vi "Comments.Add Experiment Description.vi"(7 "error in (no error)":errorcluster, 10 "Control Experiment":refnum<class "Control Experiment.lvclass">) -> (0 "error out":errorcluster, 3 "Control Experiment out":refnum<class "Control Experiment.lvclass">)   [LabVIEW 2019, in "Control Experiment.lvclass"]
uses:
  Control Experiment.lvclass
  Control Experiment.lvclass/Control Experiment.ctl
  <userlib>/LevyLab/PLYM/YAML.lvclass
panel:
  out "Experiment Description":string
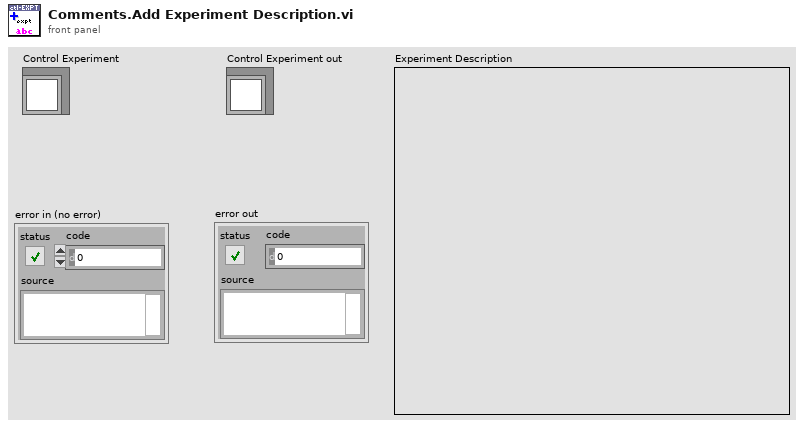
[diagram p1: front panel]
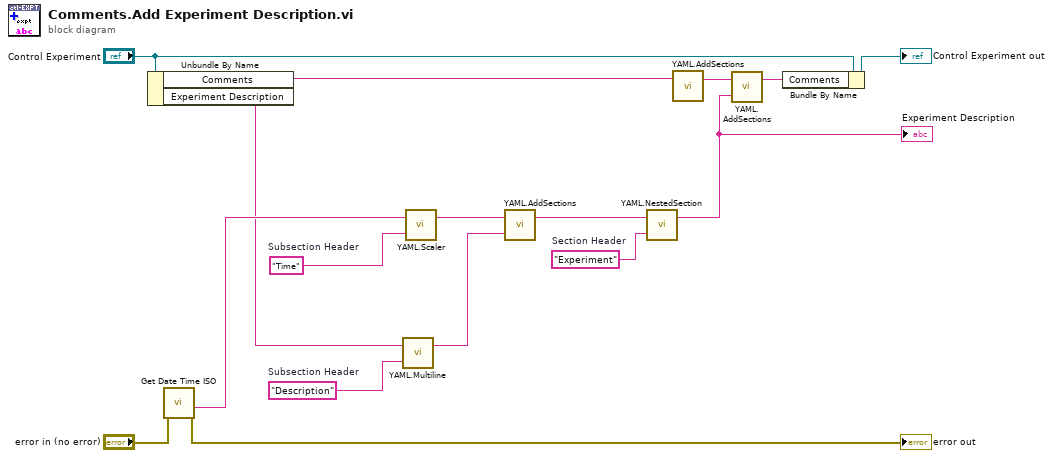
[diagram p0: block diagram]
diagram:
  w6 = "Description"  # Subsection Header
  w7 = "Time"  # Subsection Header
  w5 = "Experiment"  # Section Header
  n1 = Unbundle By Name("Control Experiment") -> ("Comments"=w3:string, "Experiment Description"=w1:string)
  n2 = call "Get Date Time ISO.vi"("error in (no error)"="error in (no error)") -> ("error out"=→"error out":errorcluster, "ISO 8601 date-time string"=w8:string)  [unwired: 8 in, 1 out]
  n3 = call <userlib>:"YAML.Multiline.vi"("Key"=w6, "Multiline"=w1) -> ("Output"=w10:string)  [unwired: 1 in]
  n4 = call <userlib>:"YAML.Scaler.vi"("Key"=w7, "Scaler"=w8) -> ("Output"=w12:string)  [unwired: 1 in]
  n5 = call <userlib>:"YAML.AddSections.vi"("Section 2"=w10, "Section 1"=w12) -> ("Output"=w9:string)  [unwired: 1 in]
  n6 = call <userlib>:"YAML.NestedSection.vi"("Section Key"=w5, "Nested Section"=w9) -> ("String"=w2:string)  [unwired: 1 in]
  "Experiment Description" <- w2
  n7 = call <userlib>:"YAML.AddSections.vi"("Section 1"=w3) -> ("Output"=w4:string)  [unwired: 2 in]
  n8 = call <userlib>:"YAML.AddSections.vi"("Section 2"=w2, "Section 1"=w4) -> ("Output"=w11:string)  [unwired: 1 in]
  n9 = Bundle By Name(cluster="Control Experiment", "Comments"=w11) -> (→"Control Experiment out":refnum<class "Control Experiment.lvclass">)
